vi "Modify Y scale marker values.vi"() -> ()   [LabVIEW 2013]
panel:
  out "Array":dbl[](array[numeric])
  out "Waveform Chart":dbl[][](graph)
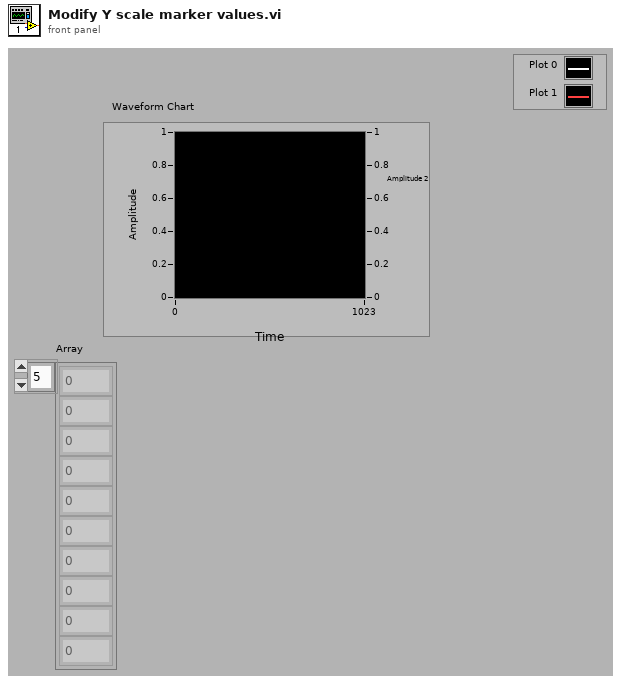
[diagram p1: front panel]
types:
  T1 = typedef "LVRangeTypeDef.ctl" = cluster{"Minimum":dbl, "Maximum":dbl, "Increment":dbl, "Minor Increment":dbl, "Start":dbl}
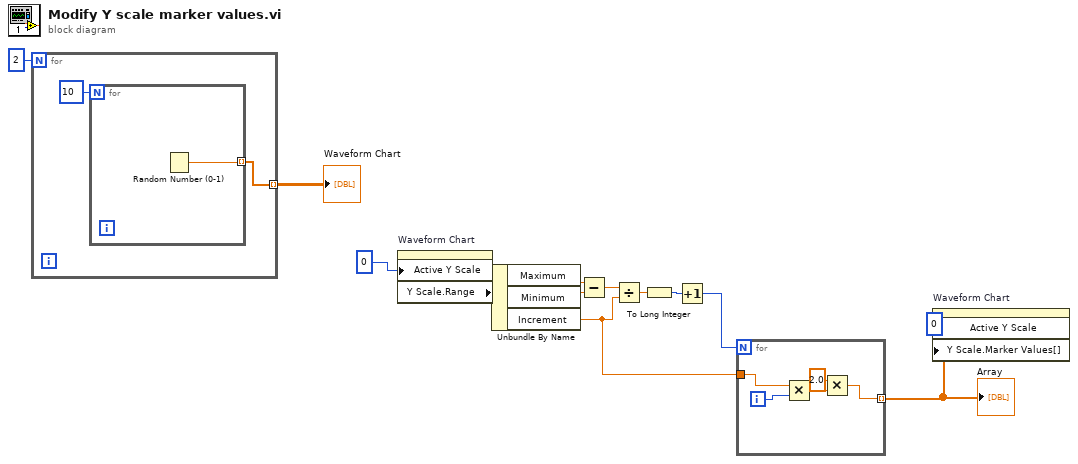
[diagram p0: block diagram]
diagram:
  n1 = for {
    N: 2 -> [_]
    tunnel: [w14] -> w12 mode=indexing
    n2 = for {
      N: 10 -> [_]
      tunnel: [w16] -> w14 mode=indexing
      n3 = Random Number (0-1)() -> (number: 0 to 1=w16:dbl)
    }
  }
  "Waveform Chart" <- w12
  n4 = property on="Waveform Chart" class="WFChart (strict)"("Active Y Scale"=0) -> ("Y Scale.Range"=w10:T1)  [unwired: 2 in, 2 out]
  n5 = Unbundle By Name(w10) -> ("Maximum"=w9:dbl, "Minimum"=w8:dbl, "Increment"=w4:dbl)
  n6 = Subtract(x=w9, y=w8) -> (x-y=w7:dbl)
  n7 = Divide(x=w7, y=w4) -> (x/y=w6:dbl)
  n8 = To Long Integer(number=w6) -> (32bit integer=w5:i32)
  n9 = Increment(x=w5) -> (x+1=w3:i32)
  n10 = for {
    N: w3 -> [_]
    tunnel: w4 -> [w20]
    tunnel: [w18] -> w1 mode=indexing
    i -> [w19]
    n11 = Multiply(x=w20, y=w19) -> (x*y=w21:dbl)
    n12 = Multiply(x=2.0, y=w21) -> (x*y=w18:dbl)
  }
  "Array" <- w1
  n13 = property on="Waveform Chart" class="WFChart (strict)"("Active Y Scale"=0, "Y Scale.Marker Values[]"=w1) -> ()  [unwired: 2 in, 2 out]
